vi "CalcGPS.vi"(0 "Grph_Stimul":waveform(dbl), 5 "Grph_Res":waveform(dbl)) -> (1 "AHV":dbl format="%0.2f", 2 "RSPV":dbl format="%0.2f", 3 "RHV":dbl format="%0.2f", 4 "AGain":dbl format="%0.2f", 6 "RGain":dbl format="%0.2f", 8 "LGain":dbl format="%0.2f", 10 "Phase":dbl, 12 "ASPV":dbl format="%0.2f", 13 "LSPV":dbl format="%0.2f", 14 "LHV":dbl format="%0.2f", 15 "Symmetry":dbl)   [LabVIEW 2013]
uses:
  <vilib>/Analysis/baseanly.llb/Mean (DBL).vi
  <vilib>/Waveform/WDTOps.llb/WDT Waveform Duration DBL.vi
  <vilib>/Waveform/WDTOps.llb/WDT Get Waveform Subset DBL.vi
  <vilib>/Analysis/NI_AALBase.lvlib
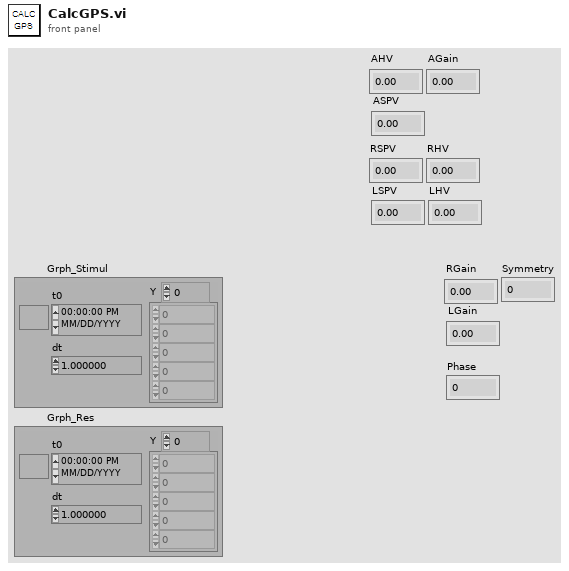
[diagram p1: front panel]
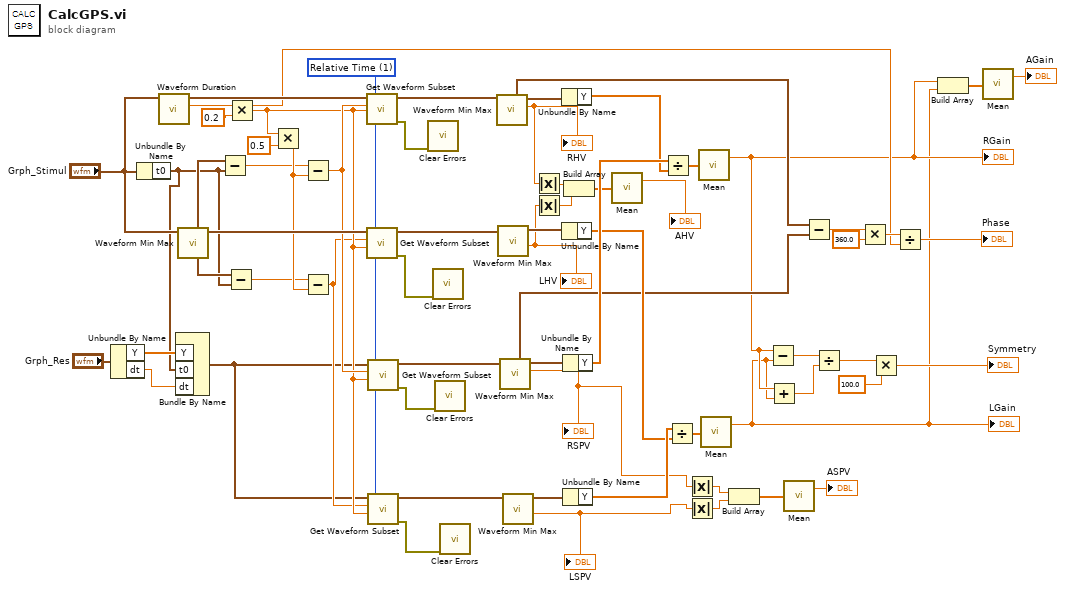
[diagram p0: block diagram]
diagram:
  w56 = u16 1 items=["Samples", "Relative Time"] ("start/duration format")
  n1 = Unbundle By Name("Grph_Res") -> ("Y"=w18:dbl[], "dt"=w17:dbl)
  n2 = Unbundle By Name("Grph_Stimul") -> ("t0"=w16:timestamp)
  n3 = call-poly <vilib>:"Waveform Duration.vi"("waveform in"="Grph_Stimul") -> ("duration"=w36:dbl, "waveform out"=w64:waveform(dbl))  [unwired: 8 in, 1 out]
  n4 = Bundle By Name("Y"=w18, "t0"=w16, "dt"=w17) -> (w15:waveform(dbl))  [unwired: 1 in]
  n5 = call <vilib>:"Waveform Min Max.vi"("waveform in"="Grph_Stimul") -> ("waveform out"=w65:waveform(dbl), "min time"=w59:timestamp, "max time"=w62:timestamp)  [unwired: 5 in, 3 out]
  n6 = Subtract(x=w62, y=w16) -> (x-y=w1:dbl)
  n7 = Subtract(x=w59, y=w16) -> (x-y=w2:dbl)
  n8 = Multiply(x=w36, y=0.2) -> (x*y=w55:dbl)
  n9 = Multiply(x=w55, y=0.5) -> (x*y=w58:dbl)
  n10 = Subtract(x=w1, y=w58) -> (x-y=w57:dbl)
  n11 = Subtract(x=w2, y=w58) -> (x-y=w54:dbl)
  n12 = call-poly <vilib>:"Get Waveform Subset.vi"("start/duration format"=w56, "duration"=w55, "start samples/time"=w57, "waveform in"=w64) -> ("error out"=w14:errorcluster, "waveform out"=w49:waveform(dbl))  [unwired: 2 in, 2 out]
  n13 = call-poly <vilib>:"Get Waveform Subset.vi"("start/duration format"=w56, "duration"=w55, "start samples/time"=w54, "waveform in"=w65) -> ("error out"=w13:errorcluster, "waveform out"=w47:waveform(dbl))  [unwired: 2 in, 2 out]
  n14 = call-poly <vilib>:"Get Waveform Subset.vi"("start/duration format"=w56, "duration"=w55, "start samples/time"=w57, "waveform in"=w15) -> ("error out"=w12:errorcluster, "waveform out"=w45:waveform(dbl))  [unwired: 2 in, 2 out]
  n15 = call-poly <vilib>:"Get Waveform Subset.vi"("start/duration format"=w56, "duration"=w55, "start samples/time"=w54, "waveform in"=w15) -> ("error out"=w11:errorcluster, "waveform out"=w43:waveform(dbl))  [unwired: 2 in, 2 out]
  n16 = call <vilib>:"Clear Errors.vi"("error in (no error)"=w14) -> ()  [unwired: 6 in, 1 out]
  n17 = call <vilib>:"Clear Errors.vi"("error in (no error)"=w13) -> ()  [unwired: 6 in, 1 out]
  n18 = call <vilib>:"Clear Errors.vi"("error in (no error)"=w12) -> ()  [unwired: 6 in, 1 out]
  n19 = call <vilib>:"Clear Errors.vi"("error in (no error)"=w11) -> ()  [unwired: 6 in, 1 out]
  n20 = call <vilib>:"Waveform Min Max.vi"("waveform in"=w49) -> ("Y max"=w9:dbl, "waveform out"=w48:waveform(dbl), "max time"=w41:timestamp)  [unwired: 5 in, 3 out]
  "RHV" <- w9
  n21 = call <vilib>:"Waveform Min Max.vi"("waveform in"=w47) -> ("Y min"=w8:dbl, "waveform out"=w46:waveform(dbl))  [unwired: 5 in, 4 out]
  "LHV" <- w8
  n22 = call <vilib>:"Waveform Min Max.vi"("waveform in"=w45) -> ("Y max"=w6:dbl, "waveform out"=w44:waveform(dbl), "max time"=w40:timestamp)  [unwired: 5 in, 3 out]
  "RSPV" <- w6
  n23 = call <vilib>:"Waveform Min Max.vi"("waveform in"=w43) -> ("Y min"=w5:dbl, "waveform out"=w42:waveform(dbl))  [unwired: 5 in, 4 out]
  "LSPV" <- w5
  n24 = Absolute Value(x=w9) -> (abs(x)=w10:dbl)
  n25 = Absolute Value(x=w8) -> (abs(x)=w7:dbl)
  n26 = Unbundle By Name(w48) -> ("Y"=w52:dbl[])
  n27 = Unbundle By Name(w46) -> ("Y"=w50:dbl[])
  n28 = Unbundle By Name(w44) -> ("Y"=w53:dbl[])
  n29 = Unbundle By Name(w42) -> ("Y"=w51:dbl[])
  n30 = Build Array(w10, w7) -> (w25:dbl[])
  n31 = call-poly <vilib>:"Mean.vi"("X"=w25) -> ("mean"=→"AHV":dbl)  [unwired: 1 out]
  n32 = Divide(x=w53, y=w52) -> (x/y=w34:dbl[])
  n33 = Divide(x=w51, y=w50) -> (x/y=w33:dbl[])
  n34 = Absolute Value(x=w6) -> (abs(x)=w4:dbl)
  n35 = Absolute Value(x=w5) -> (abs(x)=w3:dbl)
  n36 = call-poly <vilib>:"Mean.vi"("X"=w34) -> ("mean"=w27:dbl)  [unwired: 1 out]
  "RGain" <- w27
  n37 = call-poly <vilib>:"Mean.vi"("X"=w33) -> ("mean"=w26:dbl)  [unwired: 1 out]
  "LGain" <- w26
  n38 = Build Array(w4, w3) -> (w23:dbl[])
  n39 = Subtract(x=w27, y=w26) -> (x-y=w32:dbl)
  n40 = Add(x=w27, y=w26) -> (x+y=w31:dbl)
  n41 = call-poly <vilib>:"Mean.vi"("X"=w23) -> ("mean"=→"ASPV":dbl)  [unwired: 1 out]
  n42 = Subtract(x=w41, y=w40) -> (x-y=w39:dbl)
  n43 = Divide(x=w32, y=w31) -> (x/y=w30:dbl)
  n44 = Multiply(x=w39, y=360.0) -> (x*y=w37:dbl)
  n45 = Multiply(x=w30, y=100.0) -> (x*y=→"Symmetry":dbl)
  n46 = Divide(x=w37, y=w36) -> (x/y=→"Phase":dbl)
  n47 = Build Array(w27, w26) -> (w21:dbl[])
  n48 = call-poly <vilib>:"Mean.vi"("X"=w21) -> ("mean"=→"AGain":dbl)  [unwired: 1 out]
